vi "TagDB Monitor Probe.vi"(11 "TagDB":T1) -> (2 "Value String":string, 3 "Boolean":bool)   [LabVIEW 2017]
doc: "TagDB Library 2.0.1.6\nnevstop - NEVSTOP\nCopyright (c) 2018, NEVSTOP"
uses:
  TagDB/Typedef/TagDB.ctl
  TagDB/_Support/DataAccess/TagDB Ref to DVR.vi
  TagDB/_Support/Error/_[error50000]Invalid DB REF.vi
  TagDB/TagDB.lvlib
panel:
  out "Valid?":bool
  out "Name":string
  out "DataItemFlag":timestamp
  out "DataChangeFlag":timestamp
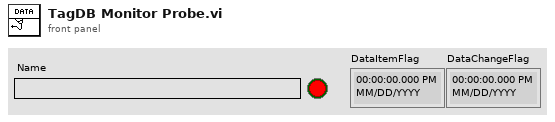
[diagram p1: front panel]
types:
  T1 = typedef "TagDB.lvlib/TagDB.ctl" = refnum<k1>
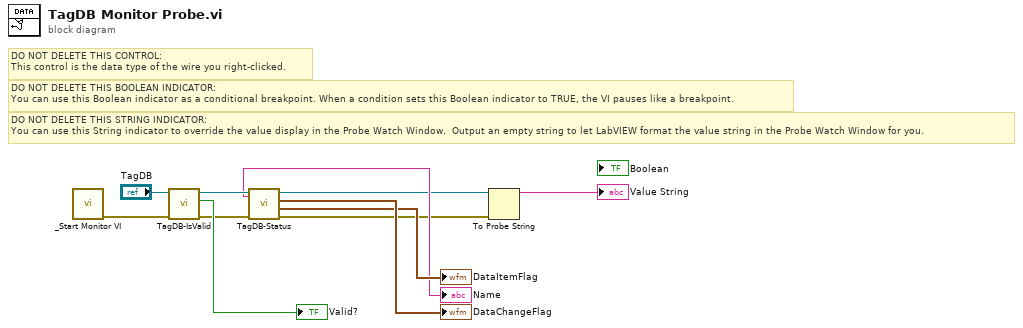
[diagram p0: block diagram]
diagram:
  # "DO NOT DELETE THIS STRING INDICATOR: \nYou can use this String indicator to override the value display in the Probe Watch Window.  Output an empty string to let LabVIEW format the value string in the Probe Watch Window for you."
  # "DO NOT DELETE THIS BOOLEAN INDICATOR: \nYou can use this Boolean indicator as a conditional breakpoint. When a condition sets this Boolean indicator to TRUE, the VI pauses like a breakpoint."
  # "DO NOT DELETE THIS CONTROL: \nThis control is the data type of the wire you right-clicked."
  n1 = call "_Start Monitor VI.vi"() -> ("error out"=w1:errorcluster)  [unwired: 11 in]
  n2 = call "TagDB-IsValid.vi"("error in (no error)"=w1, "TagDB"="TagDB") -> ("error out"=w4:errorcluster, "valid TagDB?"=→"Valid?":bool, "TagDB(dup)"=w9:T1)  [unwired: 7 in]
  n3 = call "TagDB-Status.vi"("error in (no error)"=w4, "DB Ref"=w9) -> ("error out"=w2:errorcluster, "Item Change Timestamp"=→"DataItemFlag":timestamp, "Global Change Timestamp"=→"DataChangeFlag":timestamp, "DB Ref(dup)"=w3:T1, "db name"=→"Name":string)  [unwired: 4 in, 1 out]
  n4 = To Probe String(4:w2, 7:w3) -> (3:→"Value String":string)  [unwired: 1 in, 1 out]
